vi "CalculateScanningWave.vi"() -> ()   [LabVIEW 2011]
panel:
  out "Boolean":bool
  out "Vmin":dbl
  in  "X-length 3":dbl
  in  "X-Delta 3":dbl
  in  "kineticexposure":dbl
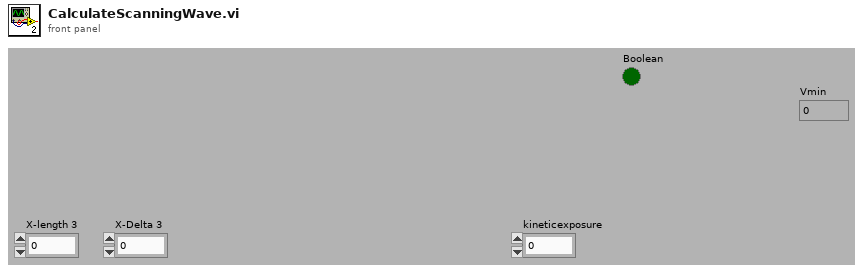
[diagram p1: front panel]
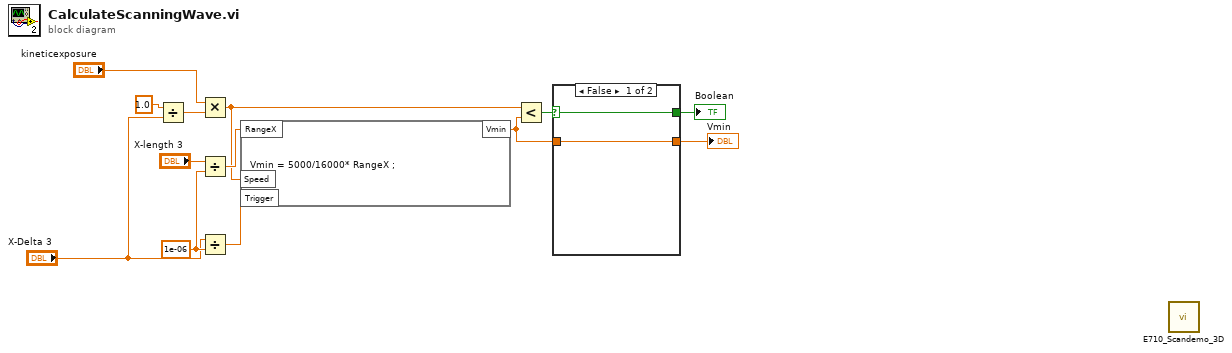
[diagram p0: block diagram]
diagram:
  w11 = 1e-06 ("y")
  n1 = Divide(x=1.0, y="X-Delta 3") -> (x/y=w7:dbl)
  n2 = Multiply(x="kineticexposure", y=w7) -> (x*y=w3:dbl)
  n3 = Divide(x="X-length 3", y=w11) -> (x/y=w12:dbl)
  n4 = Divide(x="X-Delta 3", y=w11) -> (x/y=w10:dbl)
  n5 = formula code="Vmin = 5000/16000* RangeX ;"("RangeX"=w12, "Speed"=w3, "Trigger"=w10) -> ("Vmin"=w4:dbl)
  n6 = Less?(x=w3, y=w4) -> (x < y?=w5:bool)
  n7 = case shown="False" w5 {
    selector: w5 -> [w15 w16]
    tunnel: w4 -> [w14 _]
    tunnel: [w15 w16] -> w2
    tunnel: [w14 _] -> w1
    frame False {
    }
    frame True {
    }
  }
  "Boolean" <- w2
  "Vmin" <- w1
  n8 = call "E710_Scandemo_3D.vi"() -> ()  [unwired: 28 in]
